vi "FTW-JSON-Object-Join.vi"(0 "JSON Object":refnum<class "FTW-JSON.lvclass">, 5 "JSON Object to Merge":refnum<class "FTW-JSON.lvclass">, 7 "Join Mode":T1, 11 "error in":errorcluster) -> (4 "JSON Object out":refnum<class "FTW-JSON.lvclass">, 15 "error out":errorcluster)   [LabVIEW 2015, in "FTW-JSON.lvclass"]
uses:
  FTW-JSON.lvclass
  FTW-JSON-UpdateMode.ctl
  FTW-JSON.lvclass/FTW-JSON.ctl
panel:
  # "Inputs"
  # "Outputs"
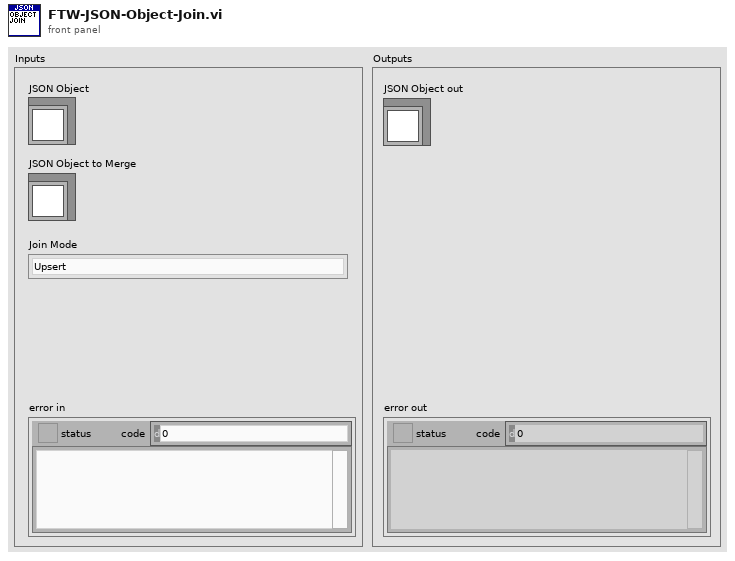
[diagram p1: front panel]
types:
  T1 = typedef "FTW-JSON.lvclass/FTW-JSON-UpdateMode.ctl" = enum16{"Upsert", "Update Only", "Insert Only"}
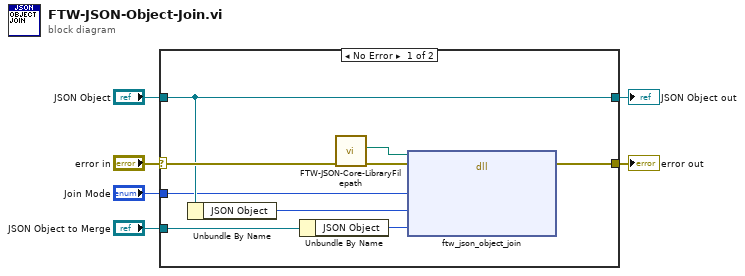
[diagram p0: block diagram]
diagram:
  n1 = case shown="No Error" "error in" {
    selector: "error in" -> [w15 w17]
    tunnel: [w12 w17] -> w6
    tunnel: [w14 w16] -> w4
    tunnel: "JSON Object" -> [w14 w16]
    tunnel: "JSON Object to Merge" -> [w13 _]
    tunnel: "Join Mode" -> [w11 _]
    frame No Error {
      n2 = Unbundle By Name(w14) -> ("JSON Object"=w8:i64)
      n3 = Unbundle By Name(w13) -> ("JSON Object"=w7:i64)
      n4 = call "FTW-JSON-Core-LibraryFilepath.vi"("error in"=w15) -> ("error out"=w10:errorcluster, "JSON Library Filepath"=w9:path)  [unwired: 9 in]
      n5 = dll-call lib="?" fn="ftw_json_object_join"(path in=w9, error in=w10, "Join Mode"=w11, "JSON Object ID"=w8, "JSON Object ID to Merge"=w7) -> (error out=w12:errorcluster)  [unwired: 5 in, 1 out]
    }
    frame Error {
    }
  }
  "error out" <- w6
  "JSON Object out" <- w4
